vi "From JSON Tree.vi"(8 "error in (no error)":errorcluster, 10 "JSON in":refnum<class "JSON Null.lvclass">, 11 "error in":refnum<class "error.lvclass">) -> (0 "error out":errorcluster, 3 "error out":refnum<class "error.lvclass">)   [LabVIEW 2015, in "error.lvclass"]
uses:
  error.lvclass
  <vilib>/National Instruments/JSON Support for LabVIEW/JSON Data Classes/JSON Datatype/JSON Null.lvclass
  error.lvclass/error.ctl
  <vilib>/National Instruments/JSON Support for LabVIEW/JSON Data Classes/JSON Helper/To More Specific Type (Object).vi
  <vilib>/National Instruments/JSON Support for LabVIEW/JSON Data Classes/JSON Object/Get Value (Numeric).vi
  <vilib>/National Instruments/JSON Support for LabVIEW/JSON Data Classes/JSON Numeric/Read value (Numeric).vi
  <vilib>/National Instruments/JSON Support for LabVIEW/JSON Data Classes/JSON Object/Get Value (String).vi
  <vilib>/National Instruments/JSON Support for LabVIEW/JSON Data Classes/JSON String/Read value (String).vi
  <vilib>/National Instruments/JSON Support for LabVIEW/JSON Data Classes/JSON Object/Get Value (JSON).vi
  <vilib>/National Instruments/JSON Support for LabVIEW/JSON Data Classes/JSON Helper/JSON Helper.lvclass
  <vilib>/National Instruments/JSON Support for LabVIEW/JSON Data Classes/JSON Basic Type/JSON Literal.lvclass
  <vilib>/National Instruments/JSON Support for LabVIEW/JSON Data Classes/JSON Numeric/JSON Numeric.lvclass
  <vilib>/National Instruments/JSON Support for LabVIEW/JSON Data Classes/JSON String/JSON String.lvclass
  <vilib>/National Instruments/JSON Support for LabVIEW/JSON Data Classes/JSON Object/JSON Object.lvclass
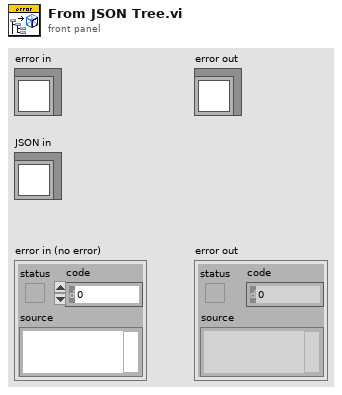
[diagram p1: front panel]
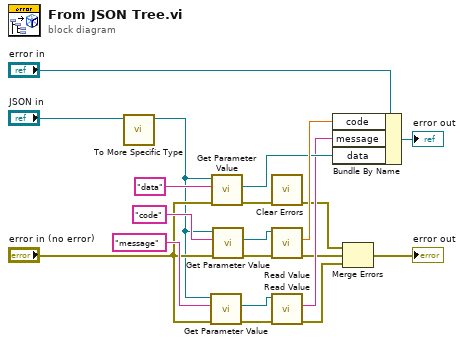
[diagram p0: block diagram]
diagram:
  n1 = call-poly <vilib>:"To More Specific Type.vi"("JSON Datatype in"="JSON in") -> ("JSON Datatype out"=w5:refnum<class "JSON Object.lvclass">)  [unwired: 9 in, 1 out]
  n2 = call-poly <vilib>:"Get Parameter Value.vi"("error in (no error)"="error in (no error)", "key"="message" ("Parameter Name"), "JSON Object in"=w5) -> ("error out"=w8:errorcluster, "value"=w3:refnum<class "JSON String.lvclass">)  [unwired: 7 in]
  n3 = call-poly <vilib>:"Get Parameter Value.vi"("error in (no error)"="error in (no error)", "key"="data" ("Parameter Name"), "JSON Object in"=w5) -> ("error out"=w2:errorcluster, "value"=w15:refnum<class "JSON Null.lvclass">)  [unwired: 7 in]
  n4 = call-poly <vilib>:"Get Parameter Value.vi"("error in (no error)"="error in (no error)", "key"="code" ("Parameter Name"), "JSON Object in"=w5) -> ("error out"=w12:errorcluster, "value"=w4:refnum<class "JSON Numeric.lvclass">)  [unwired: 7 in]
  n5 = call <vilib>:"Clear Errors.vi"("error in (no error)"=w2) -> ("error out"=w1:errorcluster)  [unwired: 5 in, 1 out]
  n6 = call-poly <vilib>:"Read Value.vi"("error in (no error)"=w12, "JSON String in"=w4) -> ("error out"=w10:errorcluster, "value"=w17:dbl)  [unwired: 8 in]
  n7 = call-poly <vilib>:"Read Value.vi"("error in (no error)"=w8, "JSON String in"=w3) -> ("error out"=w9:errorcluster, "value"=w13:string)  [unwired: 8 in]
  n8 = Bundle By Name(cluster="error in", "code"=w17, "message"=w13, "data"=w15) -> (→"error out":refnum<class "error.lvclass">)
  n9 = Merge Errors(w1, w10, w9) -> (→"error out":errorcluster)
